vi "State_machine_client.vi"() -> ()   [LabVIEW 2010]
panel:
  out "ror 1":bool
  out "boyle 1":bool
  out "Ventil 1":bool=TRUE
  out "ror 2":bool
  out "boyle 2":bool
  out "Ventil 2":bool=TRUE
  out "Server overstyring":bool
  out "Prosess stoppet":bool
  in  "Hastighet [L/s]":dbl(knob) scale=0.0..100.0
  in  "Pause prosess":bool
  out "Tilstand":T1(ring)
  in  "Fyller og tømmer":bool
  in  "STOPP programmet":bool
  out "Tank":dbl(slide) scale=0.0..1000.0
  in  "Adresse":string
  in  "Port":u16
  # "Liter med vann"
  # "Fyller"
  # "Hastighet [L/s]"
  # "Tømmer"
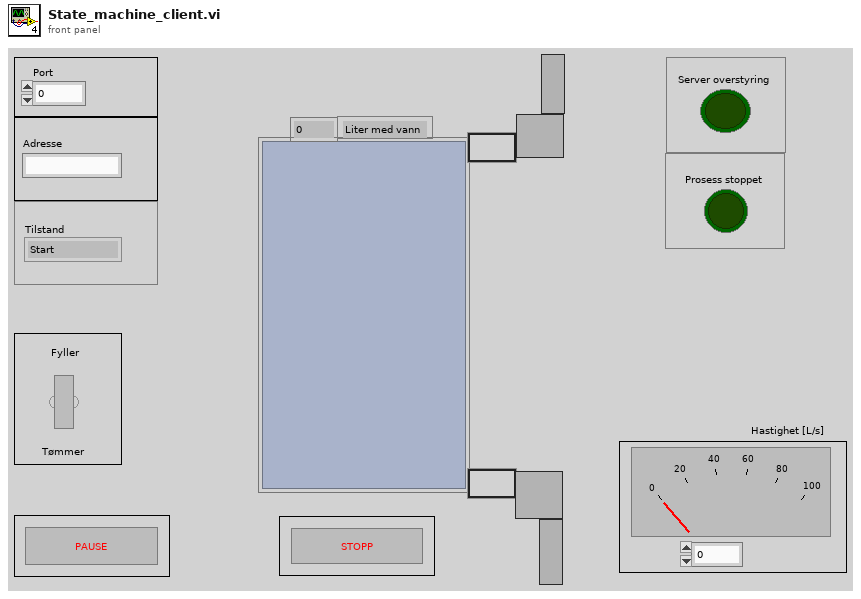
[diagram p1: front panel]
types:
  T1 = enum16{"Start", "Tomt", "Fyller", "Tømmer", "Fullt", "Stopp"}
  T2 = enum16{"Standard", "Buffered", "CRLF", "Immediate"}
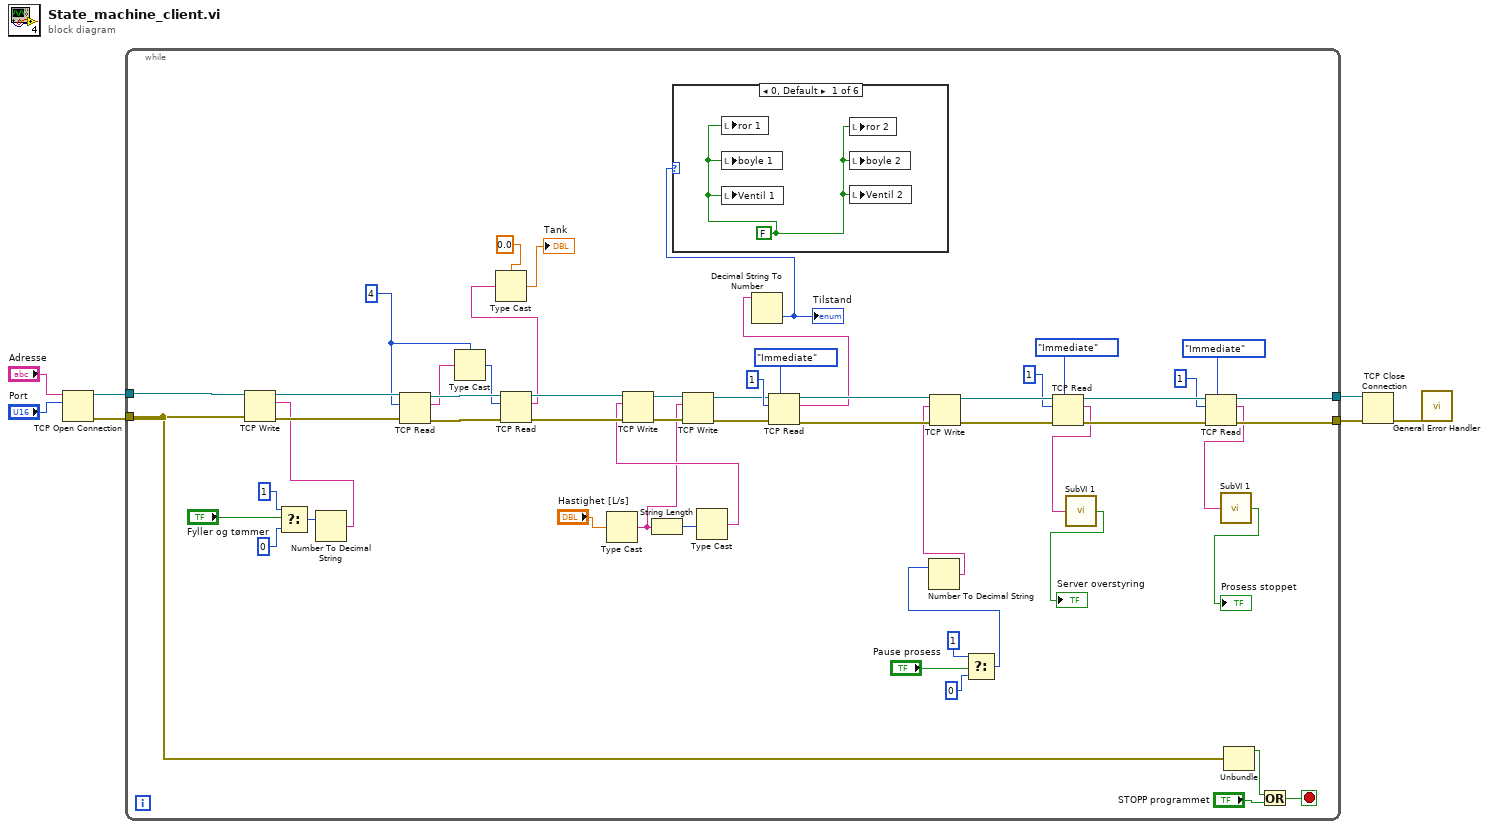
[diagram p0: block diagram]
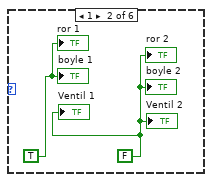
[diagram p2: hidden frame]
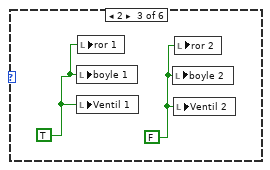
[diagram p3: hidden frame]
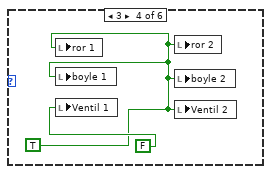
[diagram p4: hidden frame]
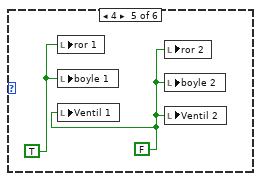
[diagram p5: hidden frame]
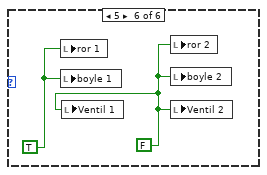
[diagram p6: hidden frame]
diagram:
  n1 = TCP Open Connection(address="Adresse", remote port or service name="Port") -> (connection ID=w7:refnum<k5>, error out=w6:errorcluster)  [unwired: 3 in]
  n2 = while {
    tunnel: w7 -> [w42]
    tunnel: w6 -> [w19]
    tunnel: [w24] -> w3
    tunnel: [w22] -> w2
    stop <- w48 stop-if-true
    w51 = 4
    n3 = Select(t=1, s="Fyller og tømmer", f=0) -> (s? t:f=w55:i32)
    n4 = Number To Decimal String(number=w55) -> (decimal integer string=w8:string)  [unwired: 1 in]
    n5 = TCP Write(connection ID=w42, data in=w8, error in (no error)=w19) -> (connection ID out=w60:refnum<k5>, error out=w59:errorcluster)  [unwired: 1 in, 1 out]
    n6 = TCP Read(connection ID=w60, bytes to read=w51, error in (no error)=w59) -> (connection ID out=w53:refnum<k5>, data out=w50:string, error out=w54:errorcluster)  [unwired: 2 in]
    n7 = Type Cast(type=w51, x=w50) -> (*(type *) &x=w52:i32)
    n8 = TCP Read(connection ID=w53, bytes to read=w52, error in (no error)=w54) -> (connection ID out=w35:refnum<k5>, data out=w18:string, error out=w40:errorcluster)  [unwired: 2 in]
    n9 = Type Cast(type=0.0, x=w18) -> (*(type *) &x=→"Tank":dbl)
    n10 = Type Cast(x="Hastighet [L/s]") -> (*(type *) &x=w15:string)  [unwired: 1 in]
    n11 = String Length(string=w15) -> (length=w33:i32)
    n12 = Type Cast(x=w33) -> (*(type *) &x=w32:string)  [unwired: 1 in]
    n13 = TCP Write(connection ID=w35, data in=w32, error in (no error)=w40) -> (connection ID out=w36:refnum<k5>, error out=w39:errorcluster)  [unwired: 1 in, 1 out]
    n14 = TCP Write(connection ID=w36, data in=w15, error in (no error)=w39) -> (connection ID out=w37:refnum<k5>, error out=w38:errorcluster)  [unwired: 1 in, 1 out]
    n15 = TCP Read(connection ID=w37, bytes to read=1, error in (no error)=w38, 7:T2."Immediate" ("mode (standard)")) -> (connection ID out=w28:refnum<k5>, data out=w11:string, error out=w43:errorcluster)  [unwired: 1 in]
    n16 = Decimal String To Number(string=w11) -> (number=w10:i32)  [unwired: 2 in, 1 out]
    "Tilstand" <- w10
    n17 = case shown="0, Default" w10 {
      frame 0, Default {
        w63 = FALSE
        n18 = local write "ror 1"(w63) -> ()
        n19 = local write "boyle 1"(w63) -> ()
        n20 = local write "Ventil 1"(w63) -> ()
        n21 = local write "ror 2"(w63) -> ()
        n22 = local write "boyle 2"(w63) -> ()
        n23 = local write "Ventil 2"(w63) -> ()
      }
      frame 1 {
        w64 = FALSE
        w65 = TRUE
        "Ventil 1" <- w64
        "boyle 1" <- w65
        "ror 1" <- w65
        "Ventil 2" <- w64
        "boyle 2" <- w64
        "ror 2" <- w64
      }
      frame 2 {
        w67 = FALSE
        w66 = TRUE
        n24 = local write "boyle 1"(w66) -> ()
        n25 = local write "Ventil 1"(w66) -> ()
        n26 = local write "ror 1"(w66) -> ()
        n27 = local write "boyle 2"(w67) -> ()
        n28 = local write "Ventil 2"(w67) -> ()
        n29 = local write "ror 2"(w67) -> ()
      }
      frame 3 {
        w68 = TRUE
        n30 = local write "ror 1"(w68) -> ()
        n31 = local write "boyle 1"(w68) -> ()
        n32 = local write "Ventil 1"(FALSE) -> ()
        n33 = local write "ror 2"(w68) -> ()
        n34 = local write "boyle 2"(w68) -> ()
        n35 = local write "Ventil 2"(w68) -> ()
      }
      frame 4 {
        w70 = FALSE
        w71 = TRUE
        n36 = local write "ror 1"(w71) -> ()
        n37 = local write "boyle 1"(w71) -> ()
        n38 = local write "Ventil 1"(w70) -> ()
        n39 = local write "ror 2"(w70) -> ()
        n40 = local write "boyle 2"(w70) -> ()
        n41 = local write "Ventil 2"(w70) -> ()
      }
      frame 5 {
        w72 = FALSE
        w73 = TRUE
        n42 = local write "ror 1"(w73) -> ()
        n43 = local write "boyle 1"(w73) -> ()
        n44 = local write "Ventil 1"(w72) -> ()
        n45 = local write "ror 2"(w72) -> ()
        n46 = local write "boyle 2"(w72) -> ()
        n47 = local write "Ventil 2"(w72) -> ()
      }
    }
    n48 = Select(t=1, s="Pause prosess", f=0) -> (s? t:f=w16:i32)
    n49 = Number To Decimal String(number=w16) -> (decimal integer string=w9:string)  [unwired: 1 in]
    n50 = TCP Write(connection ID=w28, data in=w9, error in (no error)=w43) -> (connection ID out=w29:refnum<k5>, error out=w30:errorcluster)  [unwired: 1 in, 1 out]
    n51 = TCP Read(connection ID=w29, bytes to read=1, error in (no error)=w30, 7:T2."Immediate" ("mode (standard)")) -> (connection ID out=w25:refnum<k5>, data out=w12:string, error out=w23:errorcluster)  [unwired: 1 in]
    n52 = call "SubVI 1.vi"("Input string"=w12) -> ("Output boolean"=→"Server overstyring":bool)
    n53 = TCP Read(connection ID=w25, bytes to read=1, error in (no error)=w23, 7:T2."Immediate" ("mode (standard)")) -> (connection ID out=w24:refnum<k5>, data out=w13:string, error out=w22:errorcluster)  [unwired: 1 in]
    n54 = call "SubVI 1.vi"("Input string"=w13) -> ("Output boolean"=→"Prosess stoppet":bool)
    n55 = Unbundle(w19) -> ("status"=w46:bool)  [unwired: 2 out]
    n56 = Or(x=w46, y="STOPP programmet") -> (x .or. y?=w48:bool)
  }
  n57 = TCP Close Connection(connection ID=w3, error in (no error)=w2) -> (error out=w1:errorcluster)  [unwired: 1 in, 1 out]
  n58 = call <vilib>:"General Error Handler.vi"("error in (no error)"=w1) -> ()  [unwired: 10 in, 5 out]
